vi "Pulse Output.vi"(8 "error in":errorcluster, 9 "Target":string, 11 "DIG_IO in":refnum<class "DIG_IO.lvclass">) -> (0 "error out":errorcluster, 3 "DIG_IO out":refnum<class "DIG_IO.lvclass">)   [LabVIEW 2019, in "DIG_IO.lvlib" / "DIG_IO.lvclass"]
doc: "The parent version of this VI uses an explicit time delay to pulse an output, if your device has a more effective means of pulsing the output it is preferable to use that instead of this method."
uses:
  Library/DIG_IO.lvclass
  C:/Users/Public/Documents/Development/builds/Instruments/Instruments.lvlibp/Library/Instruments.lvclass
  Library/DIG_IO.lvclass/DIG_IO.ctl
  Accessors/Read Digital.vi
  Accessors/Read Channel Names.vi
  Accessors/Read Pulse Width.vi
  builds/Instruments/Instruments.lvlibp/Private/Polymorphic/Special/Event from String.vi
  builds/Instruments/Instruments.lvlibp/Accessors/Command with Logging.vi
  builds/Instruments/Instruments.lvlibp/Library/Instruments.lvclass
  builds/Instruments/Instruments.lvlibp
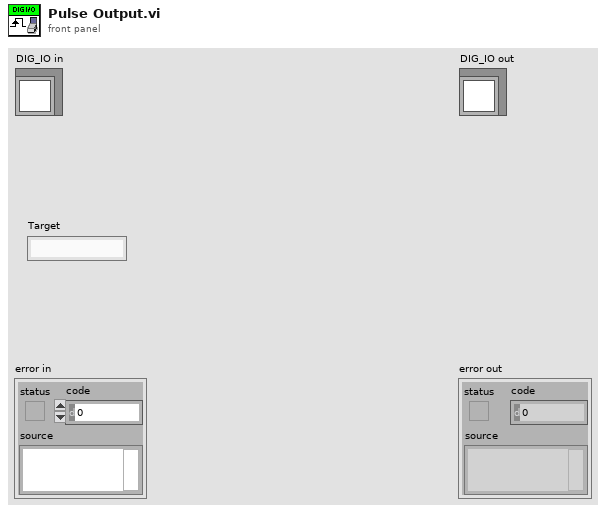
[diagram p1: front panel]
types:
  T1 = cluster{"Timestamp":timestamp, "Description":string, "Data":string}
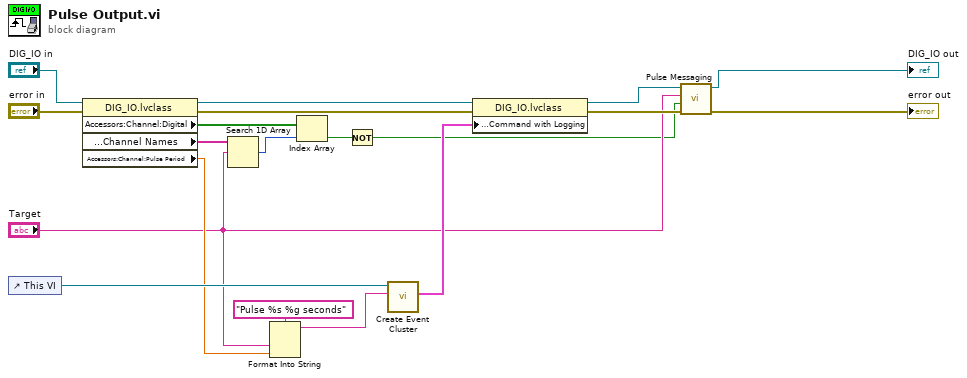
[diagram p0: block diagram]
diagram:
  n1 = control-ref of="This VI"() -> (w10:refnum<vi>)
  n2 = property class="DIG_IO.lvclass"(reference="DIG_IO in", error in="error in") -> (reference out=w12:refnum<class "DIG_IO.lvclass">, error out=w11:errorcluster, "Accessors:Channel:Digital"=w16:bool[], "Accessors:Channel:Channel Names"=w17:string[], "Accessors:Channel:Pulse Period"=w7:dbl)
  n3 = Search 1D Array(1D array=w17, element="Target") -> (index of element=w14:i32)  [unwired: 1 in]
  n4 = Format Into String(format string="Pulse %s %g seconds", "Target", w7) -> (resulting string=w9:string)  [unwired: 2 in, 1 out]
  n5 = Index Array(array=w16, index=w14) -> (element=w15:bool)
  n6 = Not(x=w15) -> (.not. x?=w1:bool)
  n7 = call-poly "Create Event Cluster.vi"("Value"=w9, "VI Refnum"=w10) -> ("Event Data"=w8:T1)  [unwired: 9 in]
  n8 = property class="DIG_IO.lvclass"(reference=w12, error in=w11, "Accessors:Logging:Command with Logging"=w8) -> (reference out=w6:refnum<class "DIG_IO.lvclass">, error out=w5:errorcluster)
  n9 = call "Pulse Messaging.vi"("error in"=w5, "Value"=w1, "Channel Name"="Target", "DIG_IO in"=w6) -> ("error out"=→"error out":errorcluster, "DIG_IO out"=→"DIG_IO out":refnum<class "DIG_IO.lvclass">)  [unwired: 6 in]
